vi "set_number_hot_cold_pixels.vi"(8 "error in (no error)":errorcluster, 9 "# hot pixels":i32 min=0 max=255, 10 "# cold pixels":i32 min=0 max=255, 11 "ColorOverlay in":refnum<class "ColorOverlay.lvclass">) -> (0 "error out":errorcluster, 3 "ColorOverlay out":refnum<class "ColorOverlay.lvclass">)   [LabVIEW 2010, in "ColorOverlay.lvclass"]
uses:
  ColorOverlay.lvclass
  ColorOverlay.lvclass/ColorOverlay.ctl
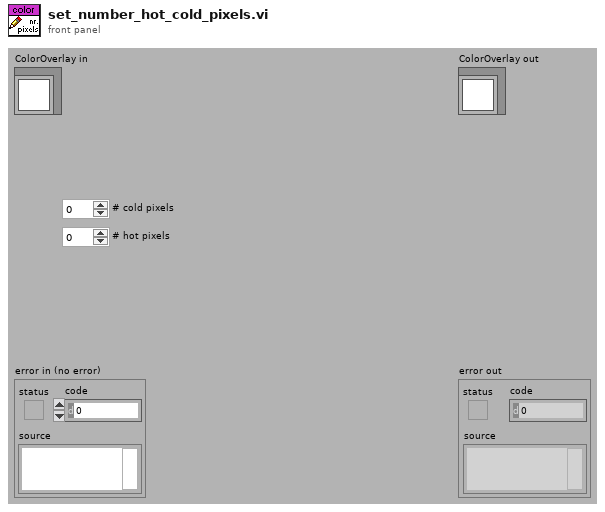
[diagram p1: front panel]
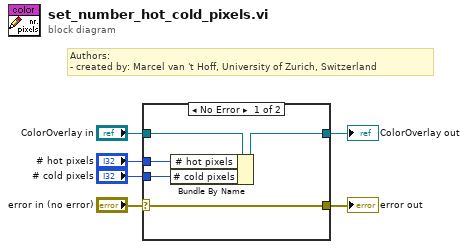
[diagram p0: block diagram]
diagram:
  # "Authors: \n- created by: Marcel van 't Hoff, University of Zurich, Switzerland"
  n1 = case shown="No Error" "error in (no error)" {
    selector: "error in (no error)" -> [w11 w13]
    tunnel: [w11 w13] -> w5
    tunnel: [w9 w12] -> w3
    tunnel: "ColorOverlay in" -> [w10 w12]
    tunnel: "# hot pixels" -> [w8 _]
    tunnel: "# cold pixels" -> [w7 _]
    frame No Error {
      n2 = Bundle By Name(cluster=w10, "# hot pixels"=w8, "# cold pixels"=w7) -> (w9:refnum<class "ColorOverlay.lvclass">)
    }
    frame Error {
    }
  }
  "error out" <- w5
  "ColorOverlay out" <- w3
